vi "Measure.vi"(6 "error in (no error)":errorcluster, 9 "Yokogawa WT2X0 in":refnum<class "Yokogawa WT2X0.lvclass">) -> (0 "error out":errorcluster, 2 "Array of Measurement":dbl[](array[numeric]), 3 "Yokogawa WT2X0 out":refnum<class "Yokogawa WT2X0.lvclass">)   [LabVIEW 2014, in "Generic Power Analyzer.lvlib" / "Yokogawa WT2X0.lvlib" / "Yokogawa WT2X0.lvclass"]
uses:
  Yokogawa WT2X0.lvclass
  Generic Power Analyzer/Generic Power Analyzer.lvclass
panel:
  out "number":dbl[](array[numeric])
  out "x^y":dbl
  out "putput":dbl
  out "input":dbl
  out "Full Array":string[][](array[string])
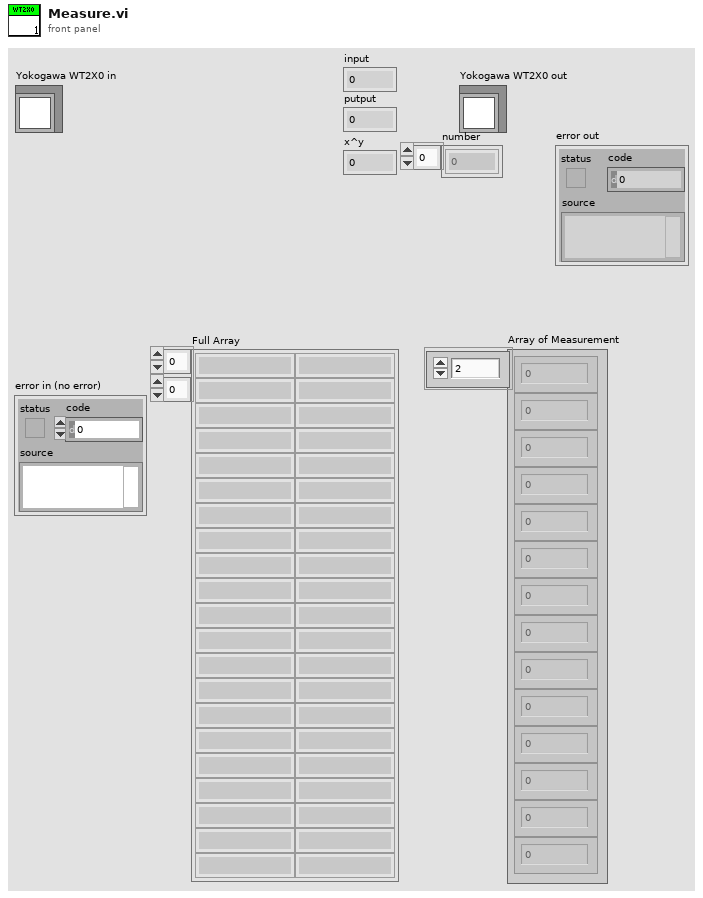
[diagram p1: front panel]
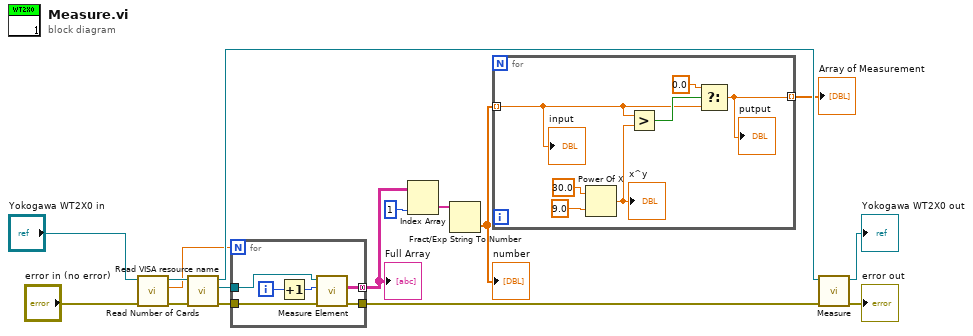
[diagram p0: block diagram]
diagram:
  n1 = call-dynamic "Read Number of Cards.vi"("error in (no error)"="error in (no error)", "Generic Instrument in"="Yokogawa WT2X0 in") -> ("error out"=w3:errorcluster, "Number of Cards"=w2:dbl, "Generic Instrument out"=w5:refnum<class "Yokogawa WT2X0.lvclass">)  [unwired: 7 in]
  n2 = call-dynamic "Read VISA resource name.vi"("error in (no error)"=w3, "Generic Instrument in"=w5) -> ("error out"=w10:errorcluster, "VISA resource name"=w9:refnum<visa-resource-name>, "Generic Instrument out"=w14:refnum<class "Yokogawa WT2X0.lvclass">)  [unwired: 7 in]
  n3 = for {
    N: w2 -> [_]
    tunnel: [w22] -> w12 mode=concatenating
    tunnel: w10 -> [w21]
    tunnel: [w20] -> w8
    tunnel: w9 -> [w19]
    i -> [w18]
    n4 = Increment(x=w18) -> (x+1=w17:i32)
    n5 = call "Measure Element.vi"("error in (no error)"=w21, "Element (1: Element 1)"=w17, "VISA resource name"=w19) -> ("error out"=w20:errorcluster, "Array"=w22:string[][])  [unwired: 6 in, 1 out]
  }
  "Full Array" <- w12
  n6 = Index Array(array=w12, index (col)=1 ("disabled index (col)")) -> (element=w11:string[])  [unwired: 1 in]
  n7 = Fract/Exp String To Number(string=w11) -> (number=w7:dbl[])  [unwired: 3 in, 1 out]
  "number" <- w7
  n8 = for {
    tunnel: w7 -> [w24] mode=indexing
    tunnel: [w23] -> w1 mode=indexing
    n9 = Power Of X(1:9.0 ("x"), 2:30.0 ("y")) -> (0:w27:dbl)
    "x^y" <- w27
    n10 = Greater?(x=w24, y=w27) -> (0:w26:bool)
    n11 = Select(t=0.0, s=w26, f=w24) -> (s? t:f=w23:dbl)
    "putput" <- w23
    "input" <- w24
  }
  "Array of Measurement" <- w1
  n12 = call-parent "Measure.vi"("error in (no error)"=w8, "Generic Power Analyzer in"=w14) -> ("error out"=→"error out":errorcluster, "Generic Power Analyzer out"=→"Yokogawa WT2X0 out":refnum<class "Yokogawa WT2X0.lvclass">)  [unwired: 5 in, 1 out]
